vi "LookAhead.vi"(8 "error in (no error)":errorcluster, 10 "Index":i32, 11 "JSON String":string) -> (0 "error out":errorcluster, 1 "TOKEN":T1)   [LabVIEW 2016, in "JSON Value.lvclass"]
uses:
  JSON Value.lvclass
  Token Type.ctl
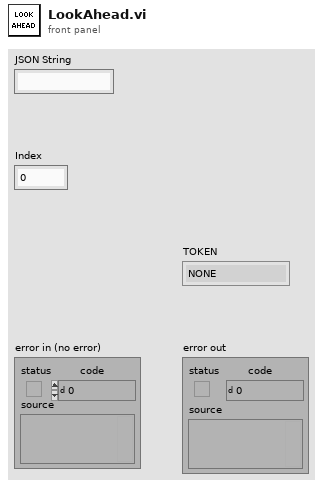
[diagram p1: front panel]
types:
  T1 = typedef "JSON Value.lvclass/Token Type.ctl" = enum8{"NONE", "CURLY_OPEN", "CURLY_CLOSE", "SQUARED_OPEN", "SQUARED_CLOSE", "COLON", "COMMA", "STRING", "NUMBER", "TRUE", "FALSE", "NULL"}
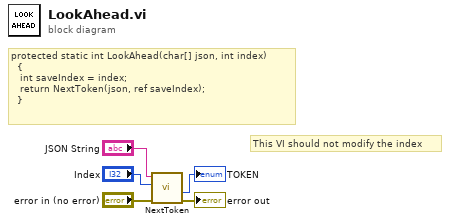
[diagram p0: block diagram]
diagram:
  # "This VI should not modify the index"
  # "protected static int LookAhead(char[] json, int index)\n\t\t{\n\t\t\tint saveIndex = index;\n\t\t\treturn NextToken(json, ref saveIndex);\n\t\t}"
  n1 = call "NextToken.vi"("error in (no error)"="error in (no error)", "Index In"="Index", "JSON String"="JSON String") -> ("error out"=→"error out":errorcluster, "TOKEN"=→"TOKEN":T1)  [unwired: 6 in, 1 out]
